vi "Convert UID To String.vi"(11 "UID":i32) -> (3 "UID string":string)   [LabVIEW 2010, in "NI_SE_Front Panel Layout.lvlib"]
uses:
  NI_SE_Front Panel Layout.lvlib
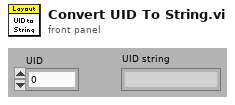
[diagram p1: front panel]
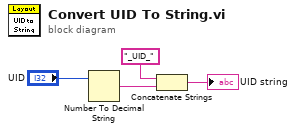
[diagram p0: block diagram]
diagram:
  n1 = Number To Decimal String(number="UID") -> (decimal integer string=w3:string)  [unwired: 1 in]
  n2 = Concatenate Strings("_UID_" ("string"), w3) -> (→"UID string":string)
